vi "To Binary.vi"(6 "byte order":T1(ring), 8 "error in (no error)":errorcluster, 11 "Type in":refnum<class "Abs_Waveform 1D.lvclass">) -> (0 "error out":errorcluster, 2 "Binary":string, 3 "Type out":refnum<class "Abs_Waveform 1D.lvclass">)   [LabVIEW 2021, in "Abs_Waveform 1D.lvclass"]
uses:
  Abs_Waveform 1D.lvclass
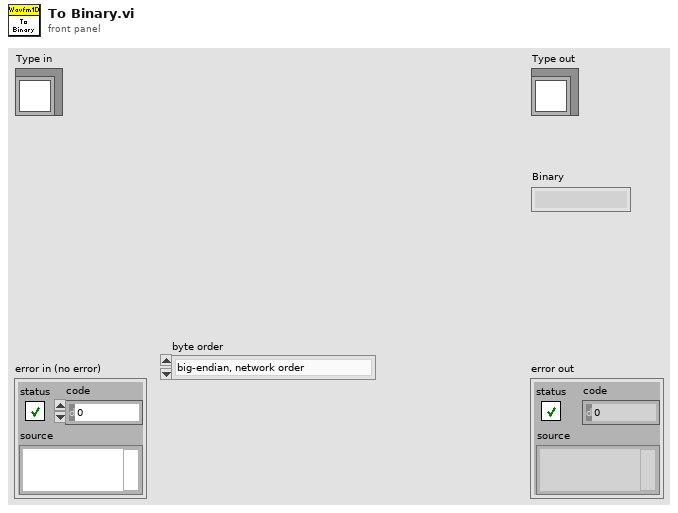
[diagram p1: front panel]
types:
  T1 = enum16{"big-endian, network order", "native, host order", "little-endian"}
  T2 = typedef "Abs_Waveform 1D.lvclass/Type.ctl" = waveform(dbl)[]
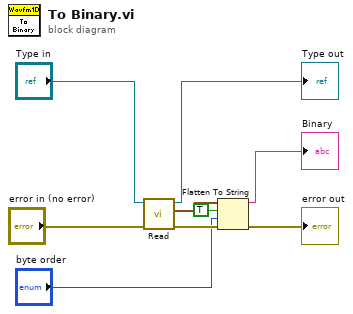
[diagram p0: block diagram]
diagram:
  n1 = call-dynamic "Read.vi"("error in (no error)"="error in (no error)", "Double Float.lvclass_340760 in"="Type in") -> ("error out"=w7:errorcluster, "Value"=w6:T2, "Double Float.lvclass_340760 out"=→"Type out":refnum<class "Abs_Waveform 1D.lvclass">)  [unwired: 7 in]
  n2 = Flatten To String(anything=w6, prepend array or string size? (T)=TRUE, byte order (0:big-endian, network order)="byte order", error in (no error)=w7) -> (data string=→"Binary":string, error out=→"error out":errorcluster)  [unwired: 1 out]
